vi "Write_Data_to_Files.vi"(2 "error in":errorcluster, 3 "Time Elapsed":string, 4 "Data in":T1={"User Name"="", "Experiment Number"=0, "Start Time"=timestamp(0 s since 1904-01-01), "Data"=[], "Step Number"=1, "Step Instructions"="", "Diagnostics"={"Langmuir Probe"=FALSE, "Rogowski 1"=FALSE, "Rogowski 2"=FALSE, "Rogowski 3"=FALSE, "B-dot 1"=FALSE, "B-dot 2"=FALSE}, "Experiment Purpose"="", "Experiment State"=enum."Off", "Systems"={"Compressed Air"=FALSE, "T-20kV Power Switch"=FALSE, "T-Rectifier"=FALSE, "Engage Interlock"=FALSE, "Ventilator"=FALSE, "Magnetron"=FALSE, "H-20kV Power Switch"=FALSE, "H-Rectifier"=FALSE, "Main Water Pump"=FALSE, "WEGA Water Pump"=FALSE, "Gas Inlet Valves"=FALSE}, "Vacuum Pressure"=0.0, "Fieldpoints"={"System Boolean Fieldpoints"={"Compressed Air"="", "T-20kV Power Switch"="", "T-Rectifier"="", "Engage Interlock"="", "Ventilator"="", "Magnetron"="", "H-20kV Power Switch"="", "H-Rectifier"="", "Main Water Pump"="", "WEGA Water Pump"="", "Gas Inlet Valves"=""}, "Step Fieldpoints"={"Exhaust Ventillator"="", "Compressed Air"="", "Water Pressure"="", "Interlock"="", "Toroidal Power Supply 1"="", "Toroidal Power Supply 2"="", "Toroidal Rectifier"="", "Helical Power Supply"="", "Helical Rectifier"="", "6kW Magnetron Standby"="", "20kW Magnetron Standby"=""}}, "Pressure History"={"Seconds into Experiment"=[], "Pressure Data"=[]}, "Time Computer Control"=[], "Toroidal Voltage Computer Control"=[], "Helical Voltage Computer Control"=[], "Toroidal Current"=[], "Toroidal Voltage"=[], "Toroidal Current Set Point"=[], "Helical Current Set Point"=[], "Helical Voltage"=[], "Helical Current"=[], "Experiment Folder"=path "", "Run Another Shot?"=FALSE}) -> (0 "error out":errorcluster, 1 "Data out":T1={"User Name"="", "Experiment Number"=0, "Start Time"=timestamp(0 s since 1904-01-01), "Data"=[], "Step Number"=1, "Step Instructions"="", "Diagnostics"={"Langmuir Probe"=FALSE, "Rogowski 1"=FALSE, "Rogowski 2"=FALSE, "Rogowski 3"=FALSE, "B-dot 1"=FALSE, "B-dot 2"=FALSE}, "Experiment Purpose"="", "Experiment State"=enum."Off", "Systems"={"Compressed Air"=FALSE, "T-20kV Power Switch"=FALSE, "T-Rectifier"=FALSE, "Engage Interlock"=FALSE, "Ventilator"=FALSE, "Magnetron"=FALSE, "H-20kV Power Switch"=FALSE, "H-Rectifier"=FALSE, "Main Water Pump"=FALSE, "WEGA Water Pump"=FALSE, "Gas Inlet Valves"=FALSE}, "Vacuum Pressure"=0.0, "Fieldpoints"={"System Boolean Fieldpoints"={"Compressed Air"="", "T-20kV Power Switch"="", "T-Rectifier"="", "Engage Interlock"="", "Ventilator"="", "Magnetron"="", "H-20kV Power Switch"="", "H-Rectifier"="", "Main Water Pump"="", "WEGA Water Pump"="", "Gas Inlet Valves"=""}, "Step Fieldpoints"={"Exhaust Ventillator"="", "Compressed Air"="", "Water Pressure"="", "Interlock"="", "Toroidal Power Supply 1"="", "Toroidal Power Supply 2"="", "Toroidal Rectifier"="", "Helical Power Supply"="", "Helical Rectifier"="", "6kW Magnetron Standby"="", "20kW Magnetron Standby"=""}}, "Pressure History"={"Seconds into Experiment"=[], "Pressure Data"=[]}, "Time Computer Control"=[], "Toroidal Voltage Computer Control"=[], "Helical Voltage Computer Control"=[], "Toroidal Current"=[], "Toroidal Voltage"=[], "Toroidal Current Set Point"=[], "Helical Current Set Point"=[], "Helical Voltage"=[], "Helical Current"=[], "Experiment Folder"=path "", "Run Another Shot?"=FALSE})   [LabVIEW 2017]
uses:
  Type_Defs/Data.ctl
  Type_Defs/Diagnostics.ctl
  Type_Defs/Systems.ctl
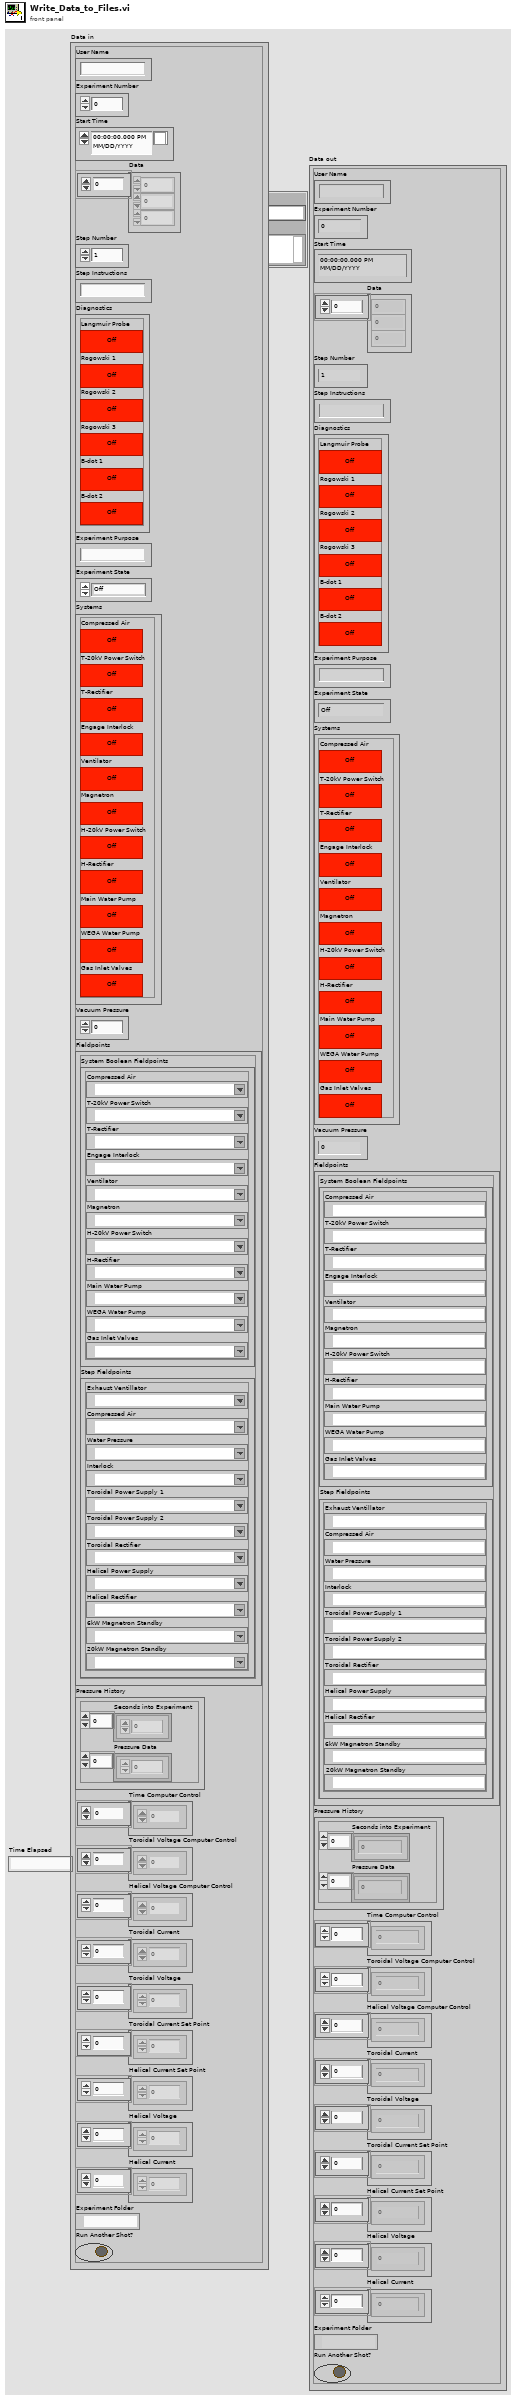
[diagram p1: front panel]
types:
  T1 = typedef "Data.ctl" = cluster{"User Name":string, "Experiment Number":i32, "Start Time":timestamp, "Data":dbl[], "Step Number":i32, "Step Instructions":string, "Diagnostics":T2, "Experiment Purpose":string, "Experiment State":enum16{"Off", "Setting Up", "Ready", "In Progress", "Shutting Down"}, "Systems":T3, "Vacuum Pressure":dbl, "Fieldpoints":cluster{"System Boolean Fieldpoints":cluster{"Compressed Air":refnum<k21>, "T-20kV Power Switch":refnum<k21>, "T-Rectifier":refnum<k21>, "Engage Interlock":refnum<k21>, "Ventilator":refnum<k21>, "Magnetron":refnum<k21>, "H-20kV Power Switch":refnum<k21>, "H-Rectifier":refnum<k21>, "Main Water Pump":refnum<k21>, "WEGA Water Pump":refnum<k21>, "Gas Inlet Valves":refnum<k21>}, "Step Fieldpoints":cluster{"Exhaust Ventillator":refnum<k21>, "Compressed Air":refnum<k21>, "Water Pressure":refnum<k21>, "Interlock":refnum<k21>, "Toroidal Power Supply 1":refnum<k21>, "Toroidal Power Supply 2":refnum<k21>, "Toroidal Rectifier":refnum<k21>, "Helical Power Supply":refnum<k21>, "Helical Rectifier":refnum<k21>, "6kW Magnetron Standby":refnum<k21>, "20kW Magnetron Standby":refnum<k21>}}, "Pressure History":cluster{"Seconds into Experiment":i32[], "Pressure Data":dbl[]}, "Time Computer Control":dbl[], "Toroidal Voltage Computer Control":dbl[], "Helical Voltage Computer Control":dbl[], "Toroidal Current":dbl[], "Toroidal Voltage":dbl[], "Toroidal Current Set Point":dbl[], "Helical Current Set Point":dbl[], "Helical Voltage":dbl[], "Helical Current":dbl[], "Experiment Folder":path, "Run Another Shot?":bool}
  T2 = typedef "Diagnostics.ctl" = cluster{"Langmuir Probe":bool, "Rogowski 1":bool, "Rogowski 2":bool, "Rogowski 3":bool, "B-dot 1":bool, "B-dot 2":bool}
  T3 = typedef "Systems.ctl" = cluster{"Compressed Air":bool, "T-20kV Power Switch":bool, "T-Rectifier":bool, "Engage Interlock":bool, "Ventilator":bool, "Magnetron":bool, "H-20kV Power Switch":bool, "H-Rectifier":bool, "Main Water Pump":bool, "WEGA Water Pump":bool, "Gas Inlet Valves":bool}
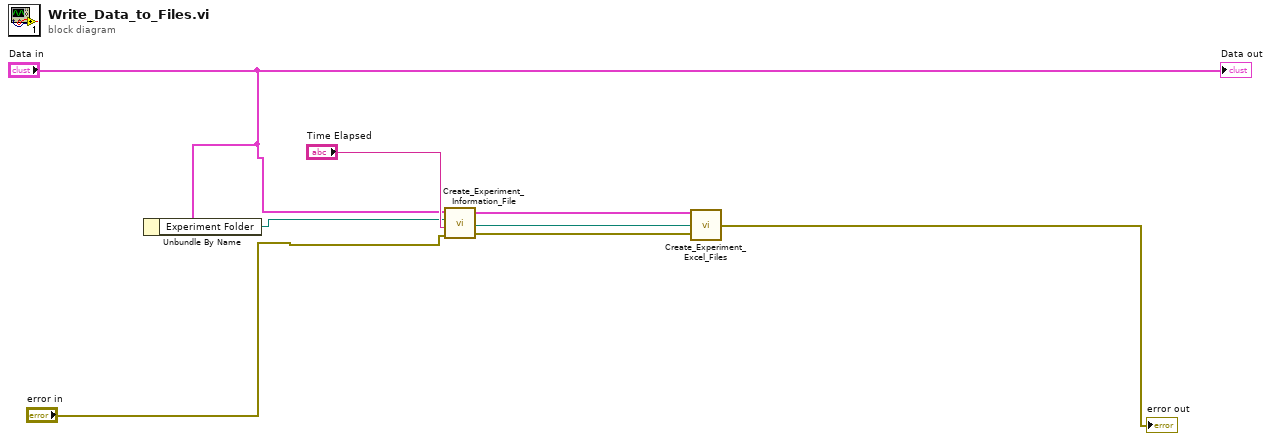
[diagram p0: block diagram]
diagram:
  n1 = Unbundle By Name("Data in") -> ("Experiment Folder"=w1:path)
  n2 = call "Create_Experiment_Information_File.vi"("error in"="error in", "Time Elapsed"="Time Elapsed", "Folder path in"=w1, "Data in"="Data in") -> ("error out"=w5:errorcluster, "Folder path out"=w6:path, "Data out"=w7:T1)
  n3 = call "Create_Experiment_Excel_Files.vi"("error in"=w5, "Folder path in"=w6, "Data in"=w7) -> ("error out"=→"error out":errorcluster)
  "Data out" <- "Data in"
